vi "Get Group.vi"(8 "error in (no error)":errorcluster, 11 "Stepper in":refnum<class "Stepper.lvclass">) -> (0 "error out":errorcluster, 2 "Group":string="p", 3 "Stepper out":refnum<class "Stepper.lvclass">)   [LabVIEW 2021, in "Stepper.lvclass"]
uses:
  Stepper.lvclass
  Stepper.lvclass/Stepper.ctl
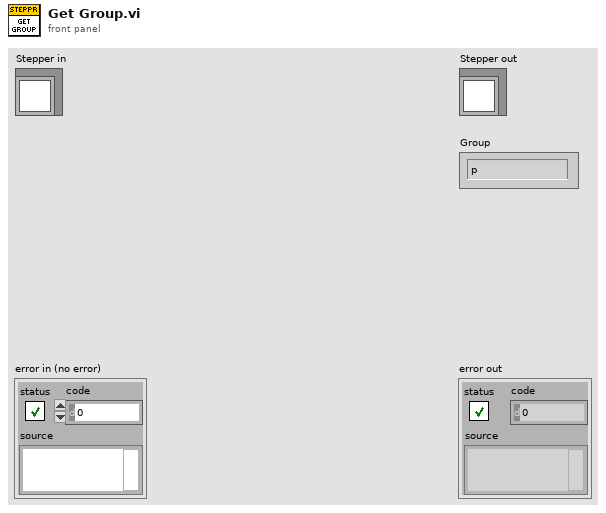
[diagram p1: front panel]
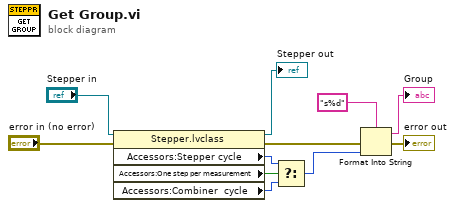
[diagram p0: block diagram]
diagram:
  n1 = property class="Stepper.lvclass"(reference="Stepper in", error in="error in (no error)") -> (reference out=→"Stepper out":refnum<class "Stepper.lvclass">, error out=w10:errorcluster, "Accessors:Stepper cycle"=w3:i32, "Accessors:One step per measurement"=w4:bool, "Accessors:Combiner  cycle"=w2:i32)
  n2 = Select(t=w3, s=w4, f=w2) -> (s? t:f=w1:i32)
  n3 = Format Into String(format string="s%d", error in=w10, w1) -> (resulting string=→"Group":string, error out=→"error out":errorcluster)  [unwired: 1 in]
